vi "PQconnectdb.vi"(8 "error in (no error)":errorcluster, 11 "conninfo":string) -> (0 "error out":errorcluster, 3 "conn":u32)   [LabVIEW 2019, in "libpqlv.lvlib"]
doc: "Makes a new connection to the database server."
uses:
  libpqlv.lvlib
  libpq.dll
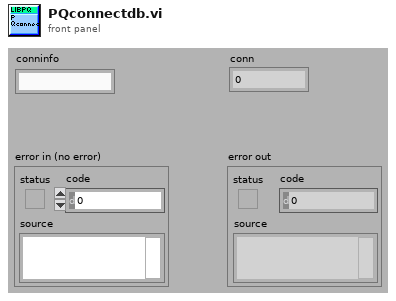
[diagram p1: front panel]
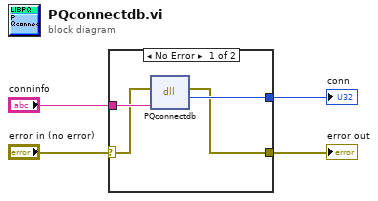
[diagram p0: block diagram]
diagram:
  n1 = case shown="No Error" "error in (no error)" {
    selector: "error in (no error)" -> [w5 w9]
    tunnel: [w6 w9] -> w3
    tunnel: [w8 _] -> w2
    tunnel: "conninfo" -> [w7 _]
    frame No Error {
      n2 = dll-call lib="libpq.*" fn="PQconnectdb"(error in=w5, "conninfo"=w7) -> (error out=w6:errorcluster, "conn"=w8:u32)  [unwired: 3 in, 1 out]
    }
    frame Error {
    }
  }
  "conn" <- w2
  "error out" <- w3
